vi "TabRefGetSubPanel.vi"(8 "error in (no error)":errorcluster, 11 "TabControl in":refnum<vi>) -> (0 "error out":errorcluster, 2 "Sub Panel":refnum<vi>, 3 "TabControl out":refnum<vi>)   [LabVIEW 2020]
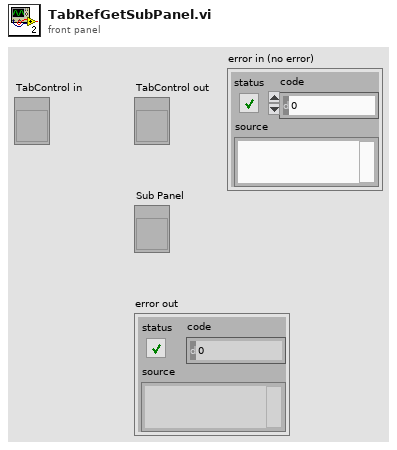
[diagram p1: front panel]
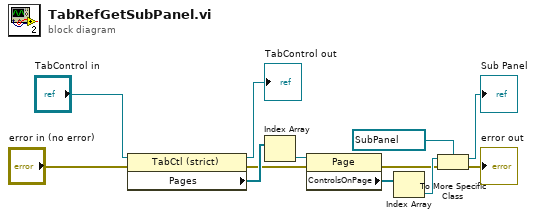
[diagram p0: block diagram]
diagram:
  n1 = property class="TabCtl (strict)"(reference="TabControl in", error in="error in (no error)") -> (reference out=→"TabControl out":refnum<vi>, error out=w2:errorcluster, "Pages"=w9:refnum<vi>[])
  n2 = Index Array(array=w9) -> (element=w10:refnum<vi>)  [unwired: 1 in]
  n3 = property class="Page"(reference=w10, error in=w2) -> (error out=w5:errorcluster, "ControlsOnPage"=w11:refnum<vi>[])  [unwired: 1 out]
  n4 = Index Array(array=w11) -> (element=w12:refnum<vi>)  [unwired: 1 in]
  n5 = To More Specific Class(target class=refnum<vi> refnum ("Sub Panel"), reference=w12, error in=w5) -> (specific class reference=→"Sub Panel":refnum<vi>, error out=→"error out":errorcluster)
